vi "Configure Probe.vi"(5 "Skew Factor (0 ms)":dbl, 6 "Coupling (0: DC)":i32(ring) items=["DC", "AC"], 7 "Units (0: Ratio)":i32(ring) items=["Ratio", "Decibel"], 8 "error in (no error)":errorcluster, 9 "Attenuation Factor (0)":dbl, 10 "Channel (1: Channel 1)":i32(ring)=1 items=["Channel 1"=1, "Channel 2"=2, "Channel 3"=3, "Channel 4"=4], 11 "VISA resource name":refnum<visa-resource-name>) -> (0 "error out":errorcluster, 3 "VISA resource name out":refnum<visa-resource-name>)   [LabVIEW 2013, in "Agilent 90000 Series.lvlib"]
doc: "Configures general settings of probe."
uses:
  Agilent 90000 Series.lvlib
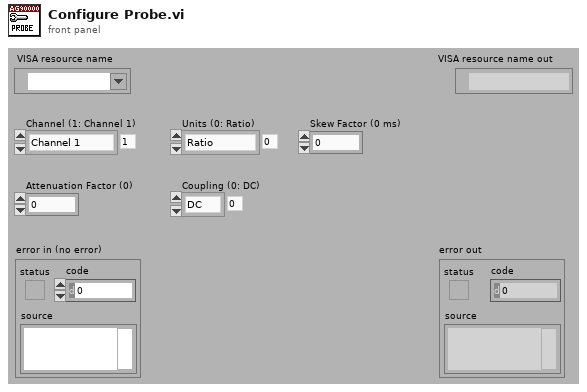
[diagram p1: front panel]
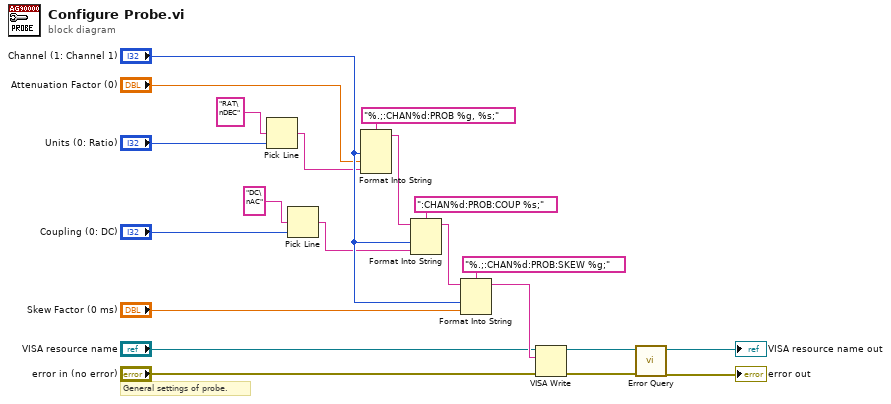
[diagram p0: block diagram]
diagram:
  # "General settings of probe."
  n1 = Pick Line(multi-line string="RAT\nDEC", line index="Units (0: Ratio)") -> (output string=w16:string)  [unwired: 1 out]
  n2 = Pick Line(multi-line string="DC\nAC", line index="Coupling (0: DC)") -> (output string=w11:string)  [unwired: 1 out]
  n3 = Format Into String(format string="%.;:CHAN%d:PROB %g, %s;", "Channel (1: Channel 1)", "Attenuation Factor (0)", w16) -> (resulting string=w13:string)  [unwired: 2 in, 1 out]
  n4 = Format Into String(format string=":CHAN%d:PROB:COUP %s;", initial string=w13, "Channel (1: Channel 1)", w11) -> (resulting string=w10:string)  [unwired: 1 in, 1 out]
  n5 = Format Into String(format string="%.;:CHAN%d:PROB:SKEW %g;", initial string=w10, "Channel (1: Channel 1)", "Skew Factor (0 ms)") -> (resulting string=w7:string)  [unwired: 1 in, 1 out]
  n6 = VISA Write(VISA resource name="VISA resource name", write buffer=w7, error in (no error)="error in (no error)") -> (VISA resource name out=w4:refnum<visa-resource-name>, error out=w3:errorcluster)  [unwired: 1 out]
  n7 = call "Error Query.vi"("error in (no error)"=w3, "VISA resource name"=w4) -> ("error out"=→"error out":errorcluster, "VISA resource name out"=→"VISA resource name out":refnum<visa-resource-name>)  [unwired: 8 out]
